vi "ES Info Data from INI.vi"(8 "error in":errorcluster, 11 "Config Refnum in":T1) -> (0 "error out":errorcluster, 3 "Config Refnum out":T1, 4 "ES_Info":T2)   [LabVIEW 2018]
uses:
  <vilib>/Utility/config.llb/Config Data RefNum.ctl
  <vilib>/ORNL/CSEISMIC DDS/CSEISMIC DDS Base/Data Types/ES_Info.ctl
  <vilib>/ORNL/CSEISMIC DDS/CSEISMIC DDS Base/Data Types/Controls/DeviceID.ctl
  <vilib>/ORNL/CSEISMIC DDS/CSEISMIC DDS Base/Data Types/Controls/EfficiencyCurve.ctl
  <vilib>/Utility/config.llb/Read Key (String).vi
  <vilib>/Utility/config.llb/Read Key (Double).vi
  <vilib>/Utility/config.llb/NI_LVConfig.lvlib
  <vilib>/ORNL/CSEISMIC DDS/CSEISMIC DDS Base/CSEISMIC DDS.lvclass
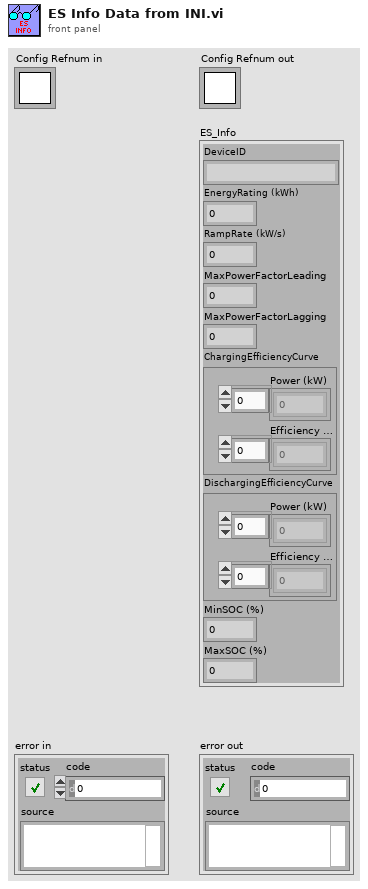
[diagram p1: front panel]
types:
  T1 = typedef "NI_LVConfig.lvlib/Config Data RefNum.ctl" = refnum<k1>
  T2 = typedef "CSEISMIC DDS.lvlib/CSEISMIC DDS.lvclass/ES_Info.ctl" = cluster{"DeviceID":T3, "EnergyRating (kWh)":dbl, "RampRate (kW/s)":dbl, "MaxPowerFactorLeading":dbl, "MaxPowerFactorLagging":dbl, "ChargingEfficiencyCurve":T4, "DischargingEfficiencyCurve":T4, "MinSOC (%)":dbl, "MaxSOC (%)":dbl}
  T3 = typedef "CSEISMIC DDS.lvlib/CSEISMIC DDS.lvclass/DeviceID.ctl" = string
  T4 = typedef "CSEISMIC DDS.lvlib/CSEISMIC DDS.lvclass/EfficiencyCurve.ctl" = cluster{"Power (kW)":dbl[], "Efficiency (%)":dbl[]}
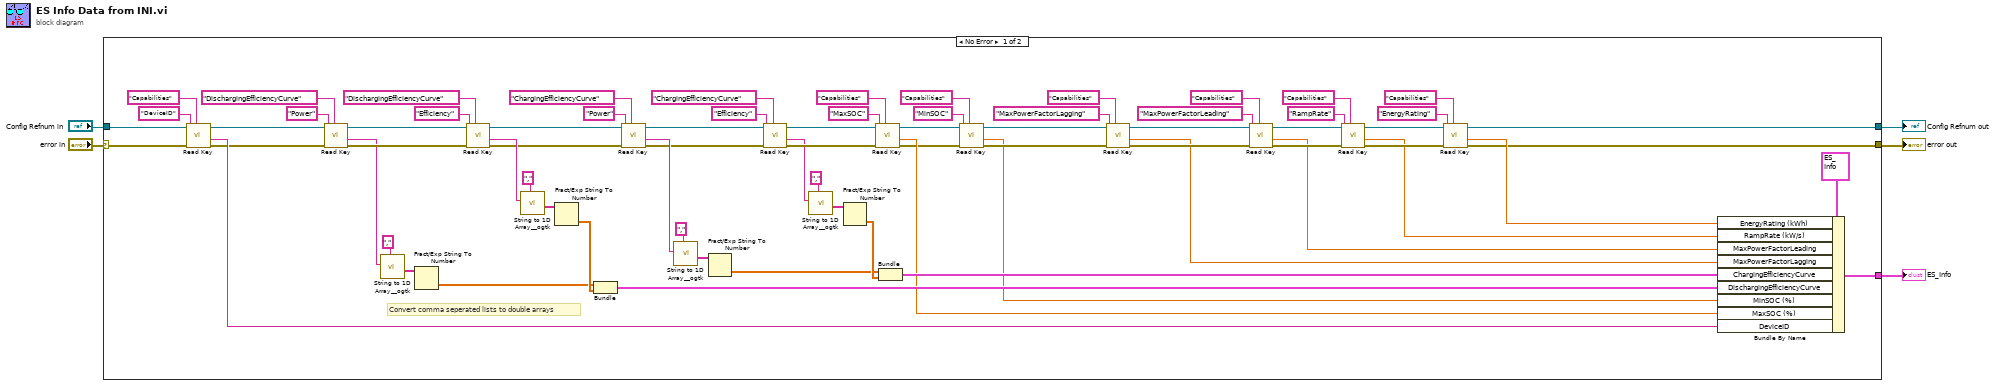
[diagram p0: block diagram]
diagram:
  n1 = case shown="No Error" "error in" {
    selector: "error in" -> [w8 w80]
    tunnel: [w6 w80] -> w5
    tunnel: [w7 w79] -> w4
    tunnel: [w72 _] -> w3
    tunnel: "Config Refnum in" -> [w9 w79]
    frame No Error {
      # "Convert comma seperated lists to double arrays"
      n2 = call-poly <vilib>:"Read Key.vi"("section"="Capabilities", "error in (no error)"=w8, "key"="DeviceID", "refnum"=w9) -> ("error out"=w10:errorcluster, "value"=w14:string, "refnum out"=w11:T1)  [unwired: 4 in, 1 out]
      n3 = call-poly <vilib>:"Read Key.vi"("section"="DischargingEfficiencyCurve", "error in (no error)"=w10, "key"="Power", "refnum"=w11) -> ("error out"=w24:errorcluster, "value"=w17:string, "refnum out"=w23:T1)  [unwired: 4 in, 1 out]
      n4 = call <userlib>:"String to 1D Array__ogtk.vi"("delimiter (Tab)"=",", "string"=w17) -> ("Array of Strings"=w19:string[])  [unwired: 9 in]
      n5 = Fract/Exp String To Number(string=w19) -> (number=w52:dbl[])  [unwired: 3 in, 1 out]
      n6 = call-poly <vilib>:"Read Key.vi"("section"="DischargingEfficiencyCurve", "error in (no error)"=w24, "key"="Efficiency", "refnum"=w23) -> ("error out"=w28:errorcluster, "value"=w39:string, "refnum out"=w27:T1)  [unwired: 4 in, 1 out]
      n7 = call <userlib>:"String to 1D Array__ogtk.vi"("delimiter (Tab)"=",", "string"=w39) -> ("Array of Strings"=w33:string[])  [unwired: 9 in]
      n8 = Fract/Exp String To Number(string=w33) -> (number=w53:dbl[])  [unwired: 3 in, 1 out]
      n9 = Bundle(w52, w53) -> (w54:cluster{dbl[], dbl[]})  [unwired: 1 in]
      n10 = call-poly <vilib>:"Read Key.vi"("section"="ChargingEfficiencyCurve", "error in (no error)"=w28, "key"="Power", "refnum"=w27) -> ("error out"=w31:errorcluster, "value"=w40:string, "refnum out"=w32:T1)  [unwired: 4 in, 1 out]
      n11 = call <userlib>:"String to 1D Array__ogtk.vi"("delimiter (Tab)"=",", "string"=w40) -> ("Array of Strings"=w36:string[])  [unwired: 9 in]
      n12 = Fract/Exp String To Number(string=w36) -> (number=w55:dbl[])  [unwired: 3 in, 1 out]
      n13 = call-poly <vilib>:"Read Key.vi"("section"="ChargingEfficiencyCurve", "error in (no error)"=w31, "key"="Efficiency", "refnum"=w32) -> ("error out"=w47:errorcluster, "value"=w41:string, "refnum out"=w46:T1)  [unwired: 4 in, 1 out]
      n14 = call <userlib>:"String to 1D Array__ogtk.vi"("delimiter (Tab)"=",", "string"=w41) -> ("Array of Strings"=w37:string[])  [unwired: 9 in]
      n15 = Fract/Exp String To Number(string=w37) -> (number=w56:dbl[])  [unwired: 3 in, 1 out]
      n16 = call-poly <vilib>:"Read Key.vi"("section"="Capabilities", "error in (no error)"=w47, "key"="MaxSOC", "refnum"=w46) -> ("error out"=w49:errorcluster, "value"=w50:dbl, "refnum out"=w48:T1)  [unwired: 4 in, 1 out]
      n17 = Bundle(w55, w56) -> (w57:cluster{dbl[], dbl[]})  [unwired: 1 in]
      n18 = call-poly <vilib>:"Read Key.vi"("section"="Capabilities", "error in (no error)"=w49, "key"="MinSOC", "refnum"=w48) -> ("error out"=w61:errorcluster, "value"=w51:dbl, "refnum out"=w60:T1)  [unwired: 4 in, 1 out]
      n19 = call-poly <vilib>:"Read Key.vi"("section"="Capabilities", "error in (no error)"=w61, "key"="MaxPowerFactorLagging", "refnum"=w60) -> ("error out"=w76:errorcluster, "value"=w68:dbl, "refnum out"=w73:T1)  [unwired: 4 in, 1 out]
      n20 = call-poly <vilib>:"Read Key.vi"("section"="Capabilities", "error in (no error)"=w76, "key"="MaxPowerFactorLeading", "refnum"=w73) -> ("error out"=w77:errorcluster, "value"=w69:dbl, "refnum out"=w74:T1)  [unwired: 4 in, 1 out]
      n21 = call-poly <vilib>:"Read Key.vi"("section"="Capabilities", "error in (no error)"=w77, "key"="RampRate", "refnum"=w74) -> ("error out"=w78:errorcluster, "value"=w70:dbl, "refnum out"=w75:T1)  [unwired: 4 in, 1 out]
      n22 = call-poly <vilib>:"Read Key.vi"("section"="Capabilities", "error in (no error)"=w78, "key"="EnergyRating", "refnum"=w75) -> ("error out"=w6:errorcluster, "value"=w71:dbl, "refnum out"=w7:T1)  [unwired: 4 in, 1 out]
      n23 = Bundle By Name(cluster=T2 {"DeviceID"="", "EnergyRating (kWh)"=0.0, "RampRate (kW/s)"=0.0, "MaxPowerFactorLeading"=0.0, "MaxPowerFactorLagging"=0.0, "ChargingEfficiencyCurve"={"Power (kW)"=[], "Efficiency (%)"=[]}, "DischargingEfficiencyCurve"={"Power (kW)"=[], "Efficiency (%)"=[]}, "MinSOC (%)"=0.0, "MaxSOC (%)"=0.0} ("ES_Info"), "EnergyRating (kWh)"=w71, "RampRate (kW/s)"=w70, "MaxPowerFactorLeading"=w69, "MaxPowerFactorLagging"=w68, "ChargingEfficiencyCurve"=w57, "DischargingEfficiencyCurve"=w54, "MinSOC (%)"=w51, "MaxSOC (%)"=w50, "DeviceID"=w14) -> (w72:T2)
    }
    frame Error {
    }
  }
  "error out" <- w5
  "Config Refnum out" <- w4
  "ES_Info" <- w3
